vi "main.vi"() -> ()   [LabVIEW 2025]
uses:
  Controls/States.ctl
  Controls/HR_Data_Structure.ctl
  Controls/Raw_Data_IN_HR.ctl
  Controls/Runner_Data_Structure.ctl
panel:
  out "XY Graph":T1(graph)
  out "BPM":cluster{"Time":timestamp[], "Bpm":i32[]}(graph)
  out "HEART RATE ZONE":string[][](array[string])
  in  "File Path":path
  out "error out":errorcluster
  in  "error in":errorcluster
  in  "Stop":bool
  in  "Save Results":bool
  in  "New Training":bool
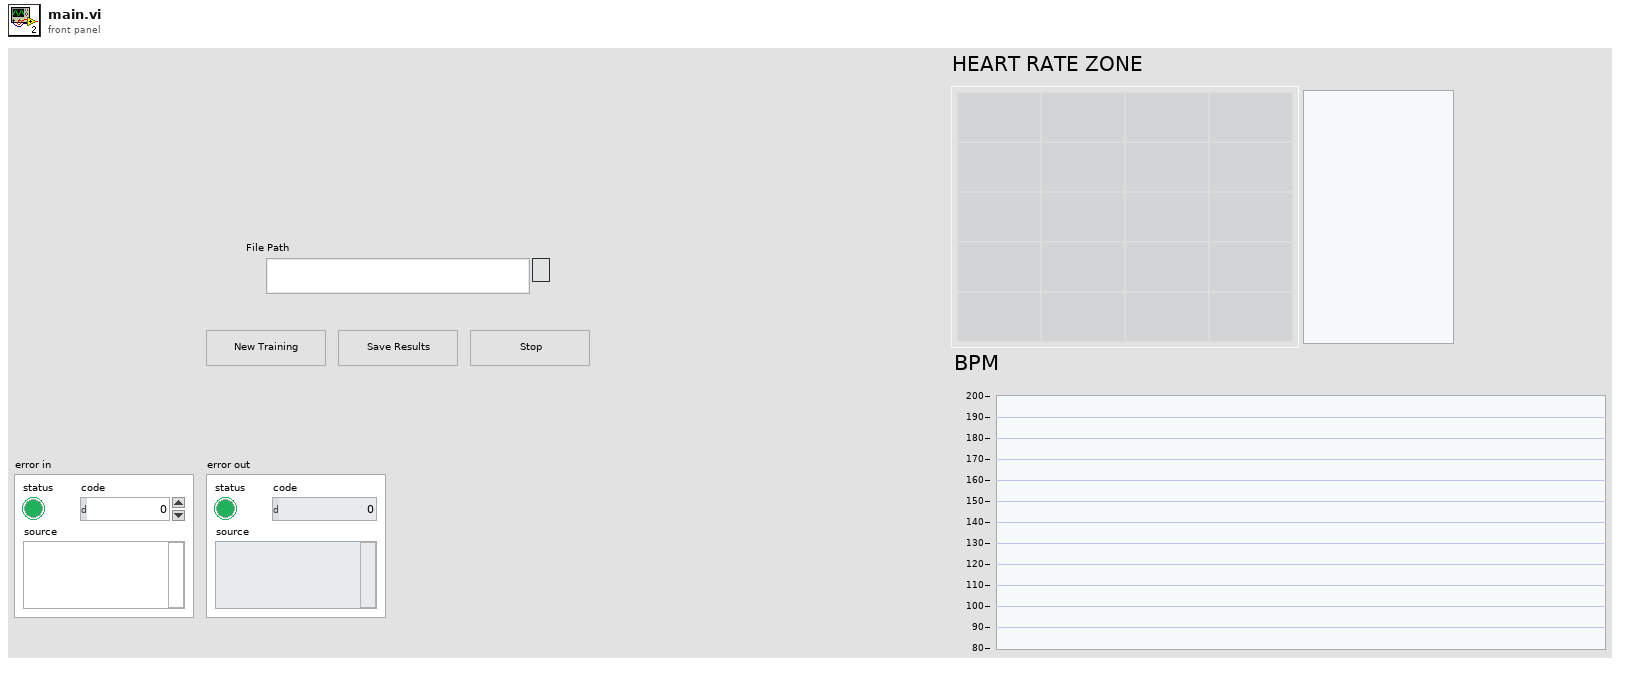
[diagram p1: front panel]
types:
  T1 = cluster{"Total Time in Zone":dbl[], "Heart Rate Zone No":dbl[]}
  T2 = typedef "HR_Data_Structure.ctl" = cluster{"HR Max":i32, "% HR MAX ":dbl[], "Raw Data":T3, "Runner's Data":T4, "HR Zone":string[][], "Total Time in Zone":dbl[], "Heart Rate Zone No":dbl[]}
  T3 = typedef "Raw_Data_IN_HR.ctl" = cluster{"Time":timestamp[], "Bpm":i32[]}
  T4 = typedef "Runner_Data_Structure.ctl" = cluster{"Name":string, "Age":i32}
  T5 = typedef "States.ctl" = enum16{"Application Error", "Init", "Idle", "Analyse New Training", "Save", "Error Handling", "Stop"}
  T6 = enum16{"open", "replace", "create", "open or create", "replace or create", "replace or create with confirmation"}
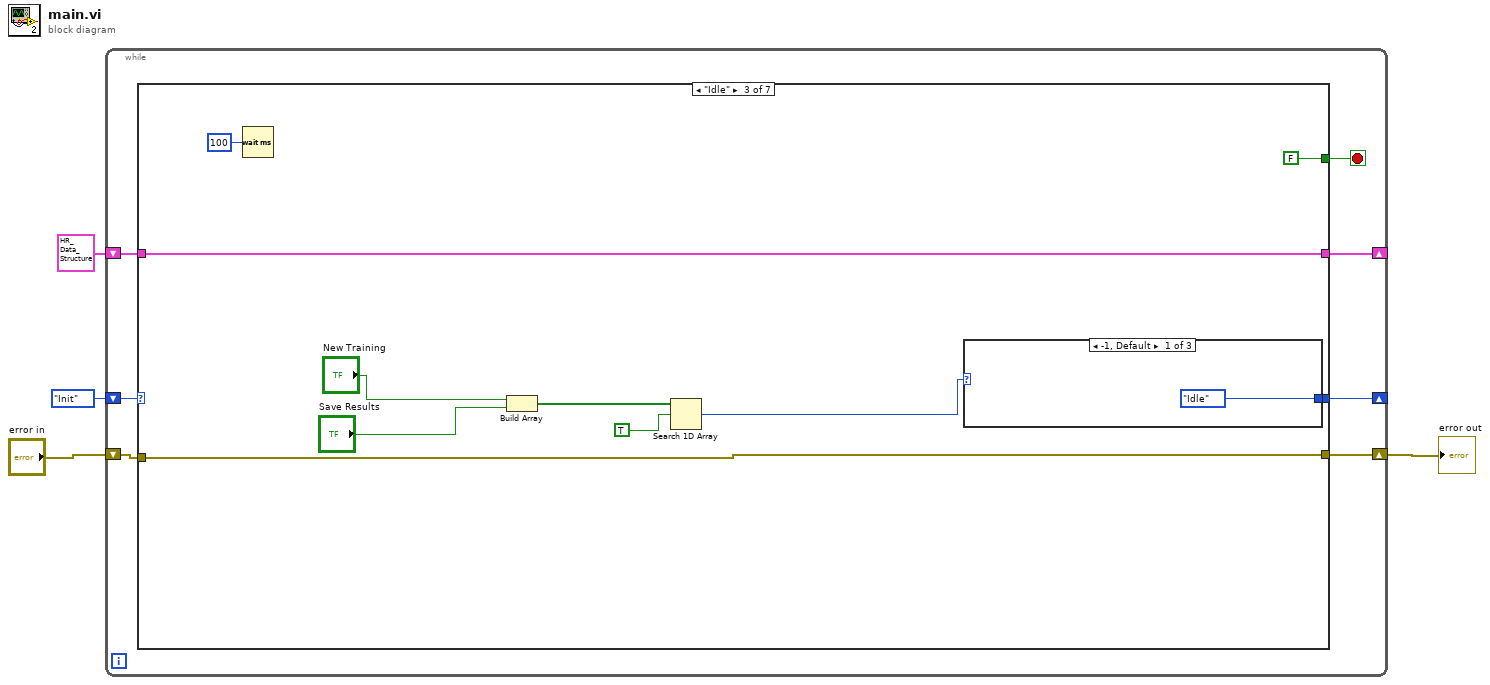
[diagram p0: block diagram]
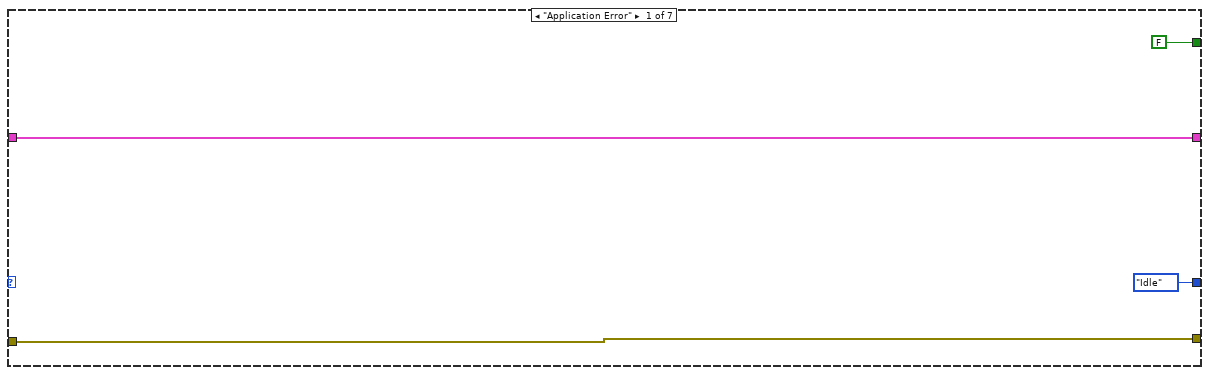
[diagram p2: hidden frame]
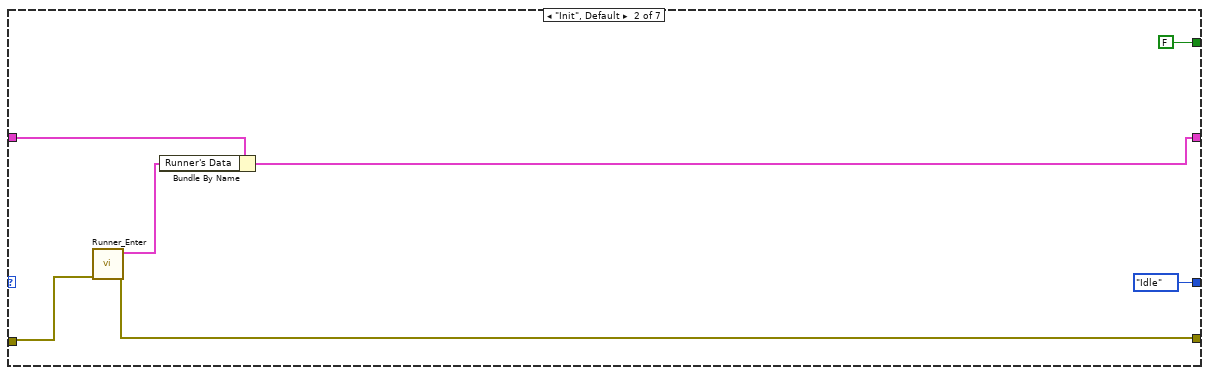
[diagram p3: hidden frame]
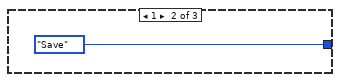
[diagram p4: hidden frame]
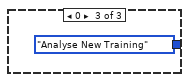
[diagram p5: hidden frame]
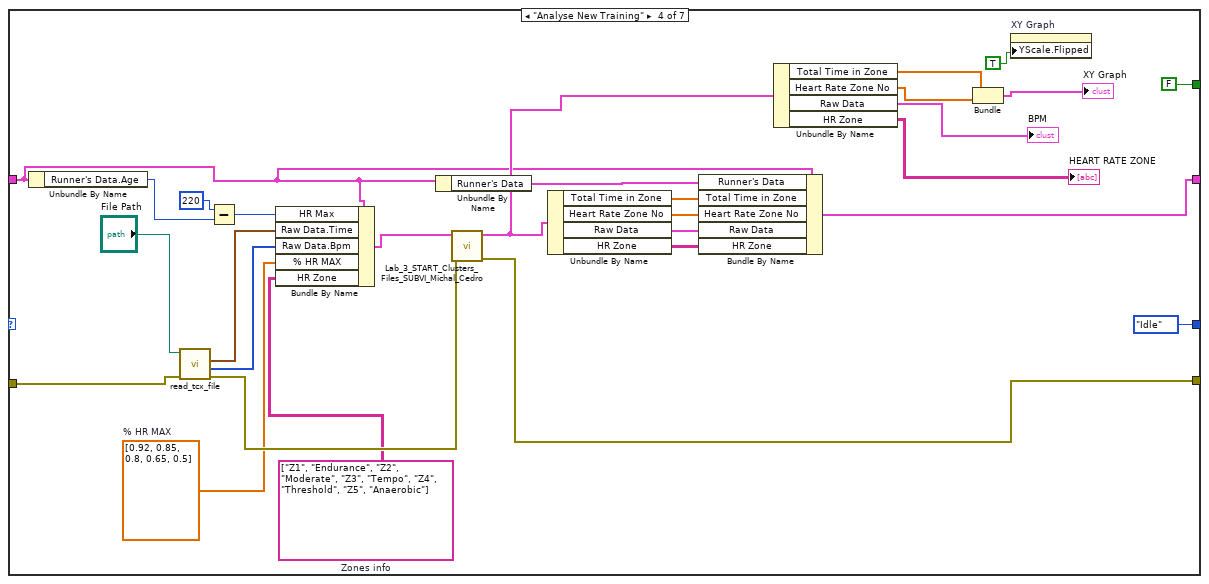
[diagram p6: hidden frame]
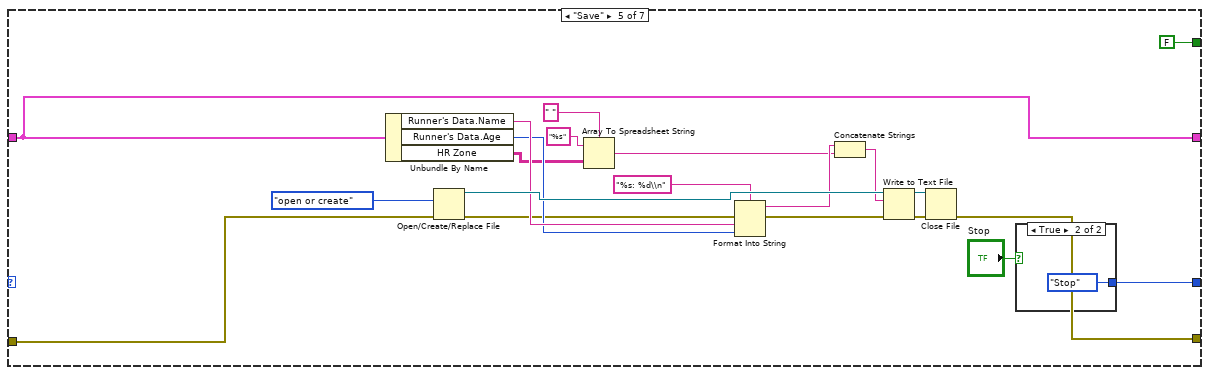
[diagram p7: hidden frame]
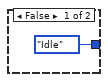
[diagram p8: hidden frame]
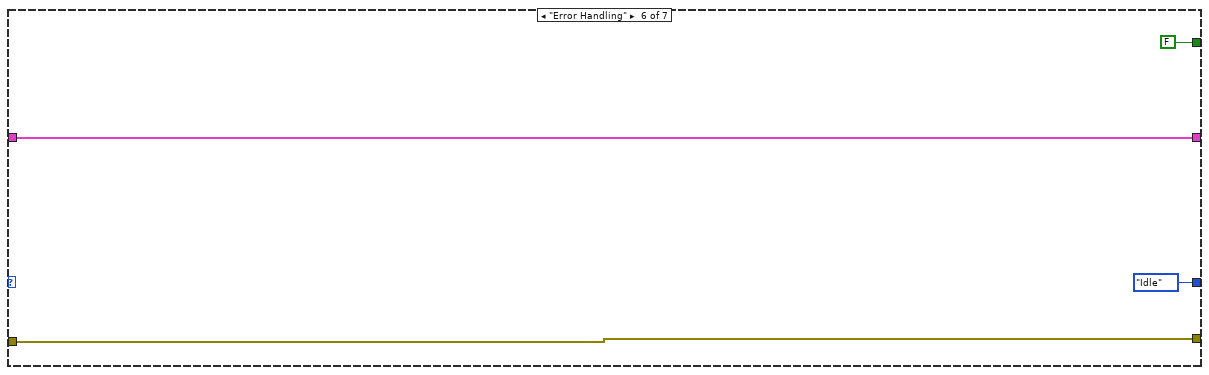
[diagram p9: hidden frame]
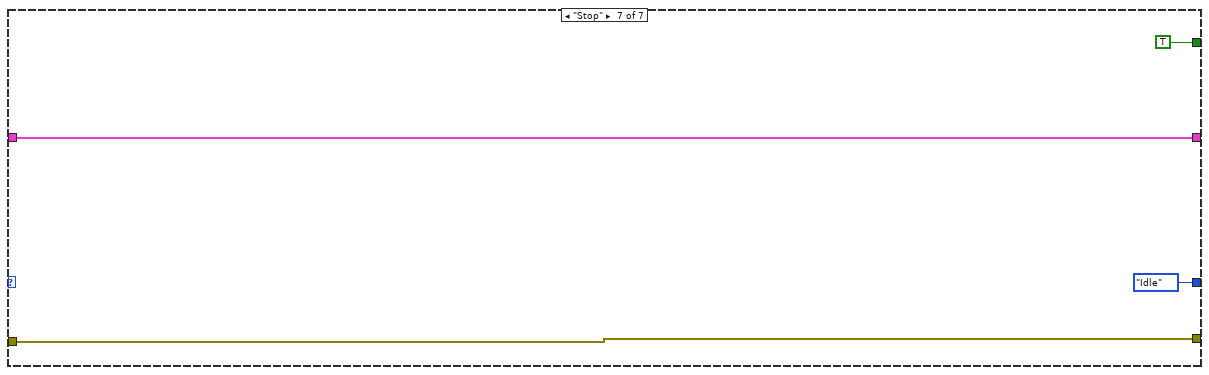
[diagram p10: hidden frame]
diagram:
  n1 = while {
    shift-right: [w11] -> _
    shift-left: States."Init" -> [w5]
    shift-right: [w8] -> _
    shift-left: T2 data[18004B] ("HR Data Structure 2") -> [w7]
    shift-right: [w9] -> w2
    shift-left: "error in" -> [w10]
    stop <- w6 stop-if-true
    n2 = case shown="\"Idle\"" w5 {
      tunnel: [States."Idle" States."Idle" w32 States."Idle" w76 States."Idle" States."Idle"] -> w11
      tunnel: w10 -> [w13 w20 w31 w50 w82 w89 w93]
      tunnel: [w13 w19 w31 w51 w79 w89 w93] -> w9
      tunnel: [w14 w18 w29 w53 w78 w90 w92] -> w8
      tunnel: w7 -> [w14 w17 w29 w36 w78 w90 w92]
      tunnel: [FALSE FALSE FALSE FALSE FALSE FALSE TRUE] -> w6
      frame "Application Error" {
      }
      frame "Init", Default {
        n3 = call "Runner_Enter.vi"("error in"=w20) -> ("error out"=w19:errorcluster, "Runner's Data OUT"=w22:T4)  [unwired: 9 in]
        n4 = Bundle By Name(cluster=w17, "Runner's Data"=w22) -> (w18:T2)
      }
      frame "Idle" {
        n5 = Wait (ms)(milliseconds to wait=u32 100) -> ()  [unwired: 1 out]
        n6 = Build Array("New Training", "Save Results") -> (w25:bool[])
        n7 = Search 1D Array(1D array=w25, element=TRUE) -> (index of element=w23:i32)  [unwired: 1 in]
        n8 = case shown="-1, Default" w23 {
          tunnel: [States."Idle" States."Save" States."Analyse New Training"] -> w32
          frame -1, Default {
          }
          frame 1 {
          }
          frame 0 {
          }
        }
      }
      frame "Analyse New Training" {
        w44 = string[][] [["Z1", "Endurance"], ["Z2", "Moderate"], ["Z3", "Tempo"], ["Z4", "Threshold"], ["Z5", "Anaerobic"]]  # Zones info
        w45 = dbl[] [0.92, 0.85, 0.8, 0.65, 0.5]  # % HR MAX
        n9 = Unbundle By Name(w36) -> ("Runner's Data.Age"=w62:i32)
        n10 = call "read_tcx_file.vi"("error in"=w50, "File Path"="File Path") -> ("error out"=w49:errorcluster, "Time"=w46:timestamp[], "Bpm"=w47:i32[])  [unwired: 7 in]
        n11 = Subtract(x=220, y=w62) -> (x-y=w60:i32)
        n12 = Bundle By Name(cluster=w36, "HR Max"=w60, "Raw Data.Time"=w46, "Raw Data.Bpm"=w47, "% HR MAX"=w45, "HR Zone"=w44) -> (w52:T2)
        n13 = Unbundle By Name(w36) -> ("Runner's Data"=w58:T4)
        n14 = call "Lab_3_START_Clusters_Files_SUBVI_Michal_Cedro.vi"("Error IN"=w49, "HR Data Structure IN"=w52) -> ("error out"=w51:errorcluster, "HR Data Structure OUT"=w37:T2)  [unwired: 8 in]
        n15 = Unbundle By Name(w37) -> ("Total Time in Zone"=w57:dbl[], "Heart Rate Zone No"=w56:dbl[], "Raw Data"=w55:T3, "HR Zone"=w54:string[][])
        n16 = Bundle By Name(cluster=w36, "Runner's Data"=w58, "Total Time in Zone"=w57, "Heart Rate Zone No"=w56, "Raw Data"=w55, "HR Zone"=w54) -> (w53:T2)
        n17 = Unbundle By Name(w37) -> ("Total Time in Zone"=w39:dbl[], "Heart Rate Zone No"=w43:dbl[], "Raw Data"=→"BPM":T3, "HR Zone"=→"HEART RATE ZONE":string[][])
        n18 = Bundle("Total Time in Zone"=w39, "Heart Rate Zone No"=w43) -> (→"XY Graph":T1)  [unwired: 1 in]
        n19 = property on="XY Graph" class="XYGraph (strict)"("YScale.Flipped"=TRUE) -> ()  [unwired: 2 in, 2 out]
      }
      frame "Save" {
        n20 = Unbundle By Name(w78) -> ("Runner's Data.Name"=w73:string, "Runner's Data.Age"=w72:i32, "HR Zone"=w69:string[][])
        n21 = Open/Create/Replace File(error in=w82, operation (0:open)=T6."open or create") -> (refnum out=w83:refnum<file>, error out=w71:errorcluster)  [unwired: 4 in, 1 out]
        n22 = Array To Spreadsheet String(delimiter (Tab)=" ", array=w69, 3:"%s" ("format string")) -> (spreadsheet string=w67:string)
        n23 = Format Into String(format string="%s: %d\\n", error in=w71, w73, w72) -> (resulting string=w68:string, error out=w70:errorcluster)  [unwired: 1 in]
        n24 = Concatenate Strings(w68, w67) -> (w66:string)
        n25 = Write to Text File(file (use dialog)=w83, text=w66, error in=w70) -> (refnum out=w81:refnum<file>, error out=w80:errorcluster)  [unwired: 1 in, 1 out]
        n26 = Close File(refnum=w81, error in=w80) -> (error out=w79:errorcluster)  [unwired: 1 out]
        n27 = case shown="True" "Stop" {
          tunnel: [States."Idle" States."Stop"] -> w76
          frame False {
          }
          frame True {
          }
        }
      }
      frame "Error Handling" {
      }
      frame "Stop" {
      }
    }
  }
  "error out" <- w2
